vi "Launcher.vi"   [LabVIEW 2017]
doc: "This is ATM launcher. This VI initializes intermodule communication. It executes Initialization API of all modules. It start all moduls. This is the most TOP of all top level VIs.\n\nThis is state machine architecture to keep block diargam clean and divided into parts.\n\nEach module is separate thread. \n[Covers: SI1] \n[Covers: SI2] \n\n-------------\nMade by:\nAnna Kozio³\n2014/09/08"
uses:
  Private controls/#TD_Launcher_States_Enum.ctl
types:
  T1 = typedef "#TD_Launcher_States_Enum.ctl" = enum16{"ERROR_Default", "InitApp", "InitErrorHandling", "InitIntermoduleCommunication", "InitModules", "RunParallelTask", "CloseIntermoduleCommunication", "StopApp"}
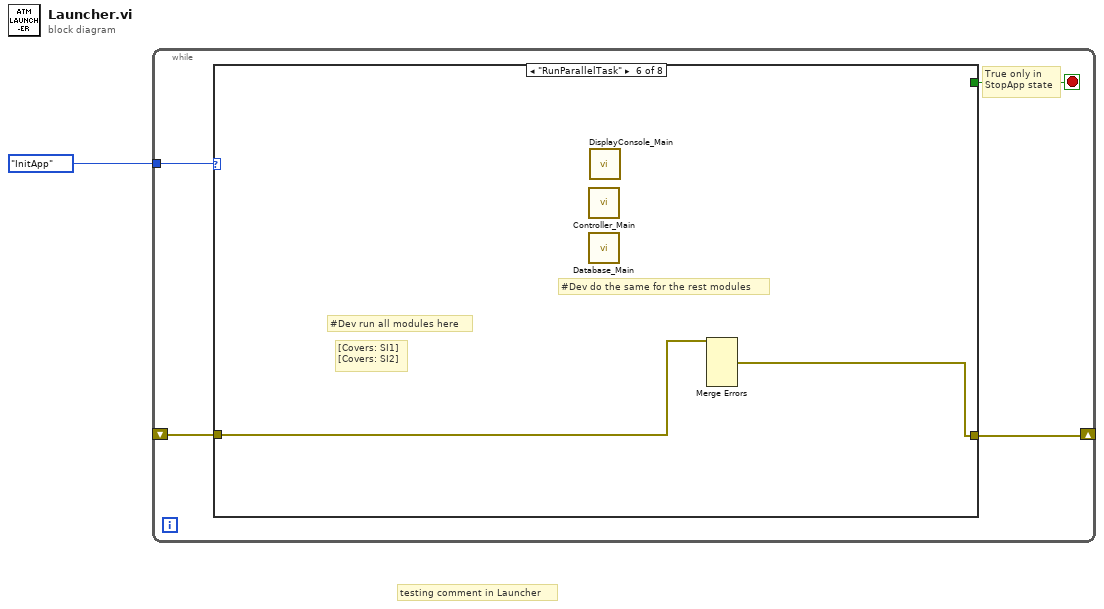
[diagram p0: block diagram]
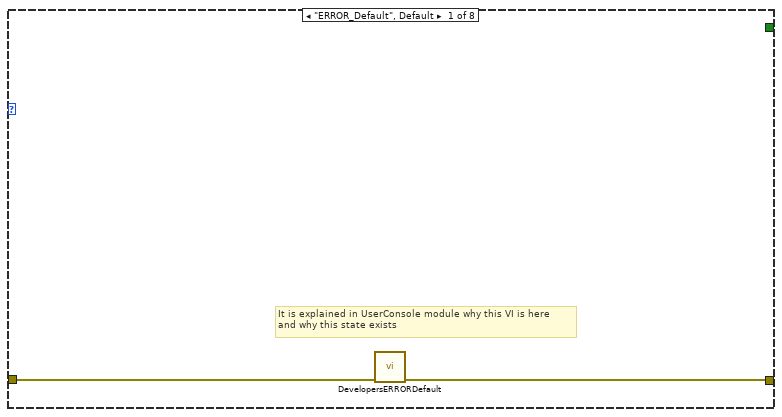
[diagram p2: hidden frame]
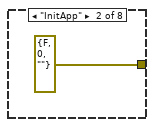
[diagram p3: hidden frame]
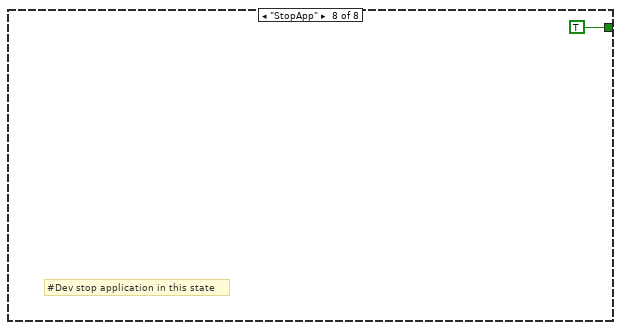
[diagram p8: hidden frame]
diagram:
  # "testing comment in Launcher"
  n1 = while {
    tunnel: #TD_Launcher_States_Enum."InitApp" -> [w5]
    shift-right: [w4] -> _
    shift-left: _ -> [w3]
    stop <- w2 stop-if-true
    # "True only in \nStopApp state"
    n2 = case shown="\"RunParallelTask\"" w5 {
      tunnel: [w6 errorcluster {"status"=FALSE, "code"=0, "source"=""} ("error in (no error)") w9 w10 w11 w13 w14 _] -> w4
      tunnel: w3 -> [w7 _ w9 w10 w11 w12 w14 _]
      tunnel: [_ _ _ _ _ _ _ TRUE] -> w2
      frame "ERROR_Default", Default {
        # "It is explained in UserConsole module why this VI is here \nand why this state exists"
        n3 = call "DevelopersERRORDefault.vi"("error in (no error)"=w7) -> ("error out"=w6:errorcluster)  [unwired: 10 in]
      }
      frame "InitApp" {
      }
      frame "InitErrorHandling" {
        # "#Dev init Error Handling module here"
      }
      frame "InitIntermoduleCommunication" {
        # "#Dev do this for the rest modules"
        # "#Dev init intermodule communications here"
      }
      frame "InitModules" {
        # "#Dev do the same for the rest modules"
        # "#Dev execute all modules Init API here"
      }
      frame "RunParallelTask" {
        # "#Dev do the same for the rest modules"
        # "[Covers: SI1] \n[Covers: SI2]"
        # "#Dev run all modules here"
        n4 = call "Controller_Main.vi"() -> ()  [unwired: 11 in, 1 out]
        n5 = call "Database_Main.vi"() -> ()  [unwired: 10 in, 2 out]
        n6 = call "DisplayConsole_Main.vi"() -> ()  [unwired: 11 in, 1 out]
        n7 = Merge Errors(w12) -> (w13:errorcluster)  [unwired: 5 in]
      }
      frame "CloseIntermoduleCommunication" {
        # "#Dev do the same for the rest modules"
        # "#Dev close intermodule communication here"
      }
      frame "StopApp" {
        # "#Dev stop application in this state"
      }
    }
  }
